vi "PID is complete.vi"(7 "sample length":i32=80, 8 "threshold":dbl=0.008, 9 "process variable":dbl, 10 "setpoint":dbl, 11 "PID Output":dbl) -> (2 "PID is Done?":bool, 3 "mean":dbl=0.00016497888749945157 format="%0.2f")   [LabVIEW 2017]
uses:
  <vilib>/ptbypt/NI_PtbyPt.lvlib
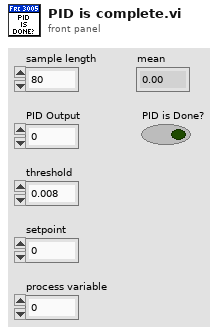
[diagram p1: front panel]
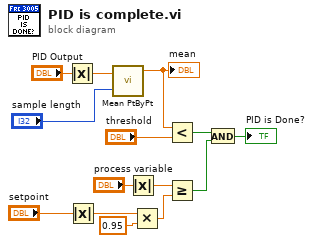
[diagram p0: block diagram]
diagram:
  n1 = Absolute Value(x="PID Output") -> (abs(x)=w3:dbl)
  n2 = Absolute Value(x="setpoint") -> (abs(x)=w1:dbl)
  n3 = call <vilib>:"Mean PtByPt.vi"("x"=w3, "sample length"="sample length") -> ("mean"=w5:dbl)  [unwired: 2 in, 1 out]
  "mean" <- w5
  n4 = Absolute Value(x="process variable") -> (abs(x)=w2:dbl)
  n5 = Multiply(x=w1, y=0.95) -> (x*y=w12:dbl)
  n6 = Less?(x=w5, y="threshold") -> (x < y?=w4:bool)
  n7 = Greater Or Equal?(x=w2, y=w12) -> (x >= y?=w14:bool)
  n8 = And(x=w4, y=w14) -> (x .and. y?=→"PID is Done?":bool)
